vi "GF_WaitTillTaskDone.vi"(1 "error in":errorcluster, 2 "timeout (sec)":dbl=10.0 format="%0.2f", 3 "task/channels in":refnum<k21>) -> (0 "error out":errorcluster)   [LabVIEW 2009]
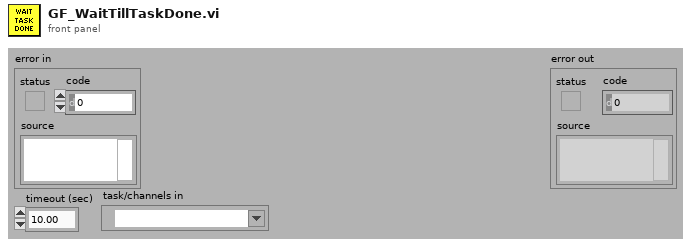
[diagram p1: front panel]
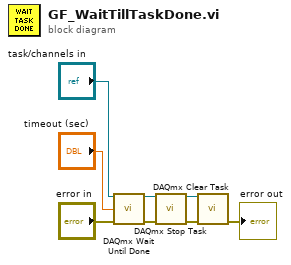
[diagram p0: block diagram]
diagram:
  n1 = call <vilib>:"DAQmx Wait Until Done.vi"("task/channels in"="task/channels in", "timeout (sec)"="timeout (sec)", "error in"="error in") -> ("task out"=w6:refnum<k21>, "error out"=w7:errorcluster)  [unwired: 11 in]
  n2 = call <vilib>:"DAQmx Stop Task.vi"("task/channels in"=w6, "error in"=w7) -> ("task out"=w5:refnum<k21>, "error out"=w8:errorcluster)  [unwired: 12 in]
  n3 = call <vilib>:"DAQmx Clear Task.vi"("task in"=w5, "error in"=w8) -> ("error out"=→"error out":errorcluster)  [unwired: 13 in]
